vi "Get Resource.vi"(8 "error in (no error)":errorcluster, 10 "name":string, 11 "Datatype group in":refnum<class "Datatype group.lvclass">) -> (0 "error out":errorcluster, 1 "resource info":variant, 2 "found":bool, 3 "Datatype group out":refnum<class "Datatype group.lvclass">)   [LabVIEW 2016, in "FPGA RM Shared API.lvlib" / "Datatype group.lvclass"]
uses:
  Datatype group.lvclass
  Datatype group.lvclass/Datatype group.ctl
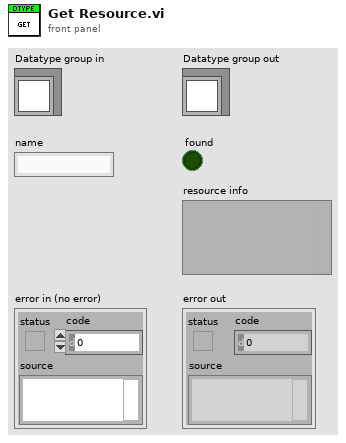
[diagram p1: front panel]
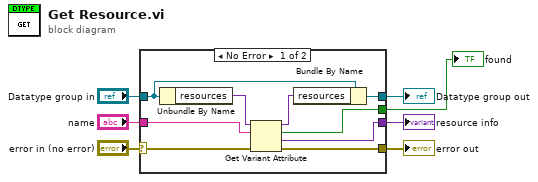
[diagram p0: block diagram]
diagram:
  n1 = case shown="No Error" "error in (no error)" {
    selector: "error in (no error)" -> [w11 w18]
    tunnel: [w10 w18] -> w6
    tunnel: [w15 w17] -> w4
    tunnel: "Datatype group in" -> [w16 w17]
    tunnel: "name" -> [w12 _]
    tunnel: [w9 _] -> w2
    tunnel: [w8 _] -> w1
    frame No Error {
      n2 = Unbundle By Name(w16) -> ("resources"=w14:variant)
      n3 = Get Variant Attribute(Variant=w14, name=w12, error in=w11) -> (duplicate Variant=w13:variant, found=w8:bool, value=w9:variant, error out=w10:errorcluster)  [unwired: 1 in]
      n4 = Bundle By Name(cluster=w16, "resources"=w13) -> (w15:refnum<class "Datatype group.lvclass">)
    }
    frame Error {
    }
  }
  "error out" <- w6
  "Datatype group out" <- w4
  "resource info" <- w2
  "found" <- w1
